vi "EXA_issueCommand_stop.vi"(8 "error in (no error)":errorcluster, 11 "command_stop_Ctl":T1) -> (0 "error out":errorcluster, 2 "function return":i32, 3 "command_stop_Ctl out":T1)   [LabVIEW 2016, in "SALLV_EXA.lvlib"]
doc: "int EXA_shm_issueCommand_stopLV(EXA_command_stopLV *command_stop_Ctl );"
uses:
  SALLV_EXA.lvlib
  DataTypes/command_stop.ctl
  SALLV_EXA.so
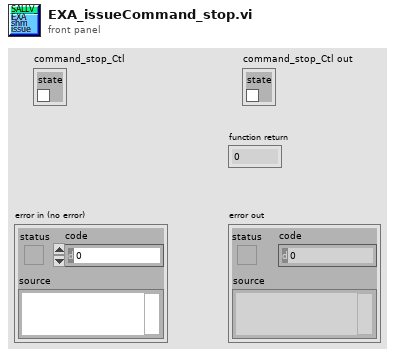
[diagram p1: front panel]
types:
  T1 = typedef "SALLV_EXA.lvlib/command_stop.ctl" = cluster{"state":bool}
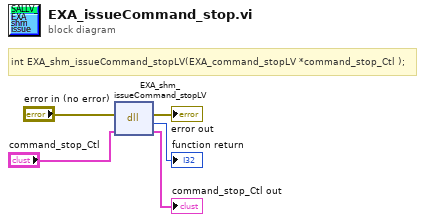
[diagram p0: block diagram]
diagram:
  # "int EXA_shm_issueCommand_stopLV(EXA_command_stopLV *command_stop_Ctl );"
  n1 = dll-call lib="home/hsundar/TCS/EXA/SALLV_EXA/SALLV_EXA.*" fn="EXA_shm_issueCommand_stopLV"(error in="error in (no error)", "command_stop_Ctl"="command_stop_Ctl") -> (error out=→"error out":errorcluster, →"function return":i32, "command_stop_Ctl"=→"command_stop_Ctl out":T1)  [unwired: 2 in, 1 out]
